vi "Write Timing Source Properties.vi"(8 "error in (no error)":errorcluster, 10 "Timing Source":T1, 11 "TimingSource in":refnum<class "TimingSource.lvclass">) -> (0 "error out":errorcluster, 3 "TimingSource out":refnum<class "TimingSource.lvclass">)   [LabVIEW 2019, in "TimingSource.lvclass"]
uses:
  TimingSource.lvclass
  XML Controls/Timing Source Properties.ctl
  XML Controls/Timing Source Source Distribution Properties.ctl
  XML Controls/Supported Targets.ctl
  XML Controls/Path Cluster.ctl
  TimingSource.lvclass/TimingSource.ctl
  VeriStand Custom Device XML Parser.lvlib
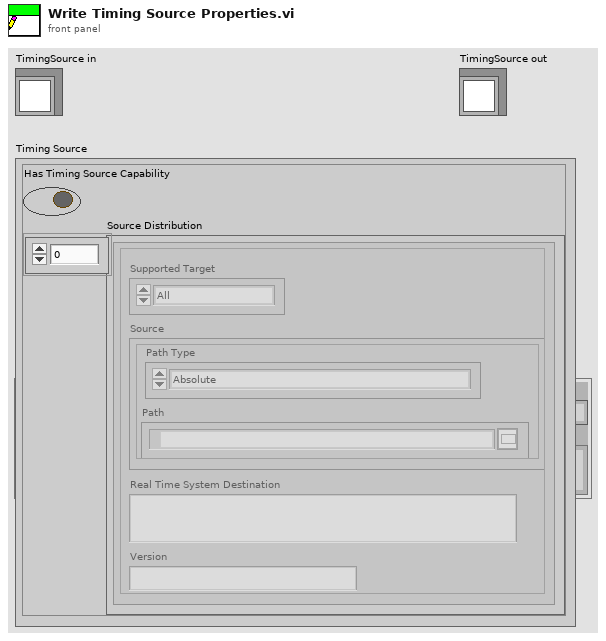
[diagram p1: front panel]
types:
  T1 = typedef "VeriStand Custom Device XML Parser.lvlib/Timing Source Properties.ctl" = cluster{"Has Timing Source Capability":bool, "Source Distribution":T2}
  T2 = typedef "VeriStand Custom Device XML Parser.lvlib/Timing Source Source Distribution Properties.ctl" = cluster{"Supported Target":T3, "Source":T4, "Real Time System Destination":string, "Version":string}[]
  T3 = typedef "VeriStand Custom Device XML Parser.lvlib/Supported Targets.ctl" = enum16{"All", "Pharlap", "VxWorks", "Windows", "Linux_32_ARM", "Linux_x64", "PharlapWindows", "PharlapVxWorks", "VxWorksWindows"}
  T4 = typedef "VeriStand Custom Device XML Parser.lvlib/Path Cluster.ctl" = cluster{"Path":path, "Path Type":enum16{"Absolute", "To Base", "To Common Doc Dir", "To Application Data Dir"}}
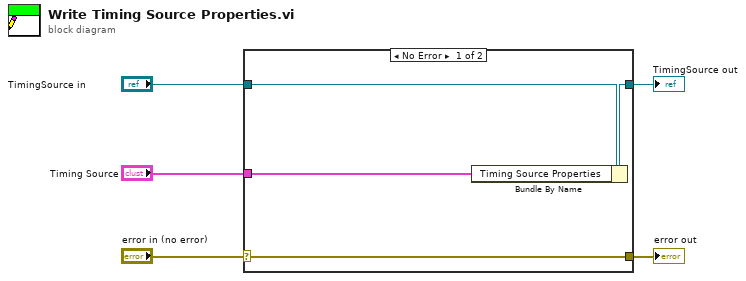
[diagram p0: block diagram]
diagram:
  n1 = case shown="No Error" "error in (no error)" {
    selector: "error in (no error)" -> [w9 w10]
    tunnel: [w9 w10] -> w4
    tunnel: [w7 w11] -> w2
    tunnel: "TimingSource in" -> [w8 w11]
    tunnel: "Timing Source" -> [w6 _]
    frame No Error {
      n2 = Bundle By Name(cluster=w8, "Timing Source Properties"=w6) -> (w7:refnum<class "TimingSource.lvclass">)
    }
    frame Error {
    }
  }
  "error out" <- w4
  "TimingSource out" <- w2
